vi "Framework_Initialize.vi"(8 "error in (no error)":errorcluster, 11 "AB_DepSourceDist in":refnum<class "AB_DepSourceDist.lvclass">) -> (0 "error out":errorcluster, 1 "helpTopics":string[](array[string]), 2 "pageTitles":string[](array[string]), 3 "AB_DepSourceDist out":refnum<class "AB_DepSourceDist.lvclass">, 4 "helpFile":string, 5 "pages":path[](array[path]))   [LabVIEW 2020, in "AB_DepSourceDist.lvclass"]
uses:
  <vilib>/AppBuilder/AB_Classes/DepSourceDist/AB_DepSourceDist.lvclass
  <vilib>/AppBuilder/AB_Classes/SourceDistribution/AB_SourceDistribution.lvclass
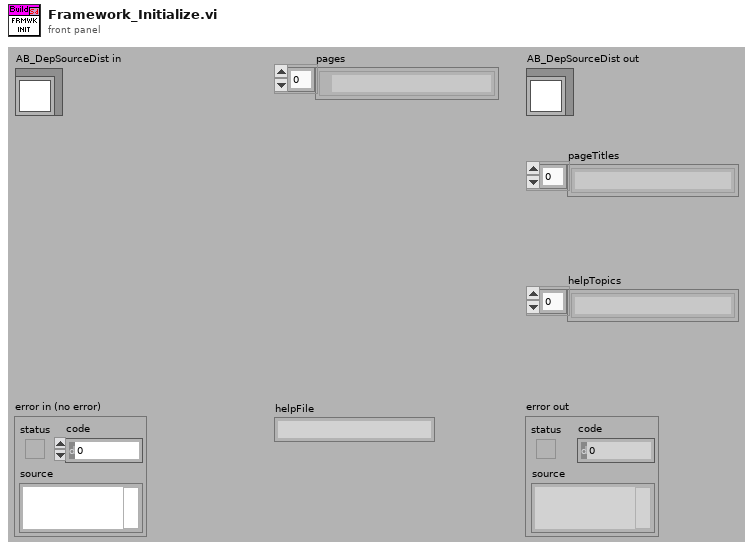
[diagram p1: front panel]
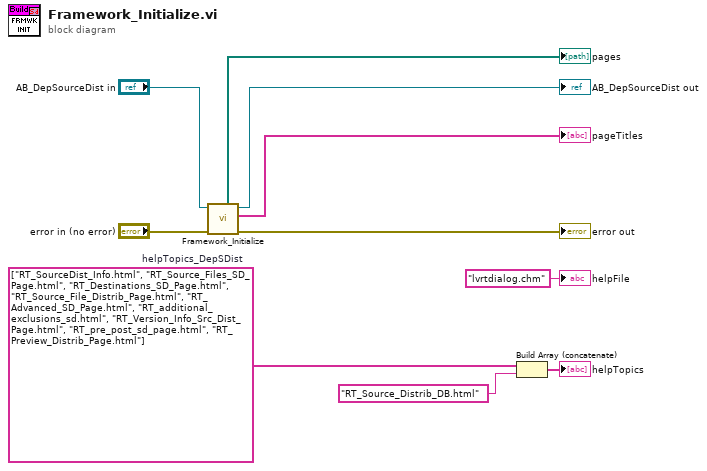
[diagram p0: block diagram]
diagram:
  w2 = string[] ["RT_SourceDist_Info.html", "RT_Source_Files_SD_Page.html", "RT_Destinations_SD_Page.html", "RT_Source_File_Distrib_Page.html", "RT_Advanced_SD_Page.html", "RT_additional_exclusions_sd.html", "RT_Version_Info_Src_Dist_Page.html", "RT_pre_post_sd_page.html", "RT_Preview_Distrib_Page.html"]  # helpTopics_DepSDist
  n1 = call-parent "Framework_Initialize.vi"("error in (no error)"="error in (no error)", "AB_SourceDistribution in"="AB_DepSourceDist in") -> ("error out"=→"error out":errorcluster, "pageTitles"=→"pageTitles":string[], "AB_SourceDistribution out"=→"AB_DepSourceDist out":refnum<class "AB_DepSourceDist.lvclass">, "pages"=→"pages":path[])  [unwired: 4 in, 2 out]
  n2 = Build Array (concatenate)(w2, "RT_Source_Distrib_DB.html" ("HTML filename")) -> (→"helpTopics":string[])
  "helpFile" <- "lvrtdialog.chm" ("helpFile")
